vi "Check_bandejas.vi"(8 "error in (no error)":errorcluster, 10 "BANDEJA ORIGEN":T2(ring), 11 "BANDEJA DESTINO":T2(ring)) -> (0 "error out":errorcluster, 2 "States_main":T1, 3 "Datos incorrectos":bool)   [LabVIEW 2019]
uses:
  TYPE'S DEF/Estados_TRASPASO.ctl
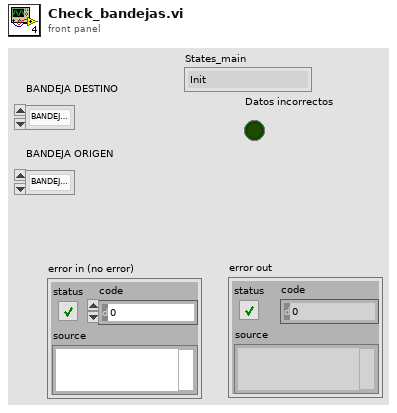
[diagram p1: front panel]
types:
  T1 = typedef "Estados_TRASPASO.ctl" = enum16{"Init", "Wait for Event", "Init refs", "Init com", "Config estacion", "Introducir valores traspaso", "Home", "Ping_Arduino", "Esperar fin movimiento", "Enviar_config_test", "Actualizar valores", "Final traspaso?", "Terminar", "Exit", "Error?"}
  T2 = enum16{"BANDEJA ENTRADA", "BANDEJA OK", "BANDEJA NOK"}
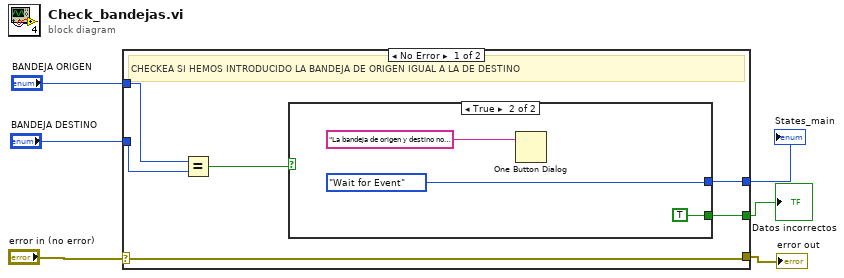
[diagram p0: block diagram]
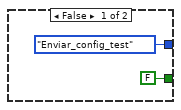
[diagram p2: hidden frame]
diagram:
  n1 = case shown="No Error" "error in (no error)" {
    selector: "error in (no error)" -> [w7 w18]
    tunnel: "BANDEJA DESTINO" -> [w12 _]
    tunnel: "BANDEJA ORIGEN" -> [w11 _]
    tunnel: [w9 _] -> w4
    tunnel: [w8 _] -> w3
    tunnel: [w7 w18] -> w1
    frame No Error {
      # "CHECKEA SI HEMOS INTRODUCIDO LA BANDEJA DE ORIGEN IGUAL A LA DE DESTINO"
      n2 = Equal?(x=w11, y=w12) -> (x = y?=w10:bool)
      n3 = case shown="True" w10 {
        tunnel: [FALSE ("Datos incorrectos") TRUE ("Datos incorrectos")] -> w9
        tunnel: [Estados_TRASPASO."Enviar_config_test" ("States_main") Estados_TRASPASO."Wait for Event" ("States_main")] -> w8
        frame False {
        }
        frame True {
          n4 = One Button Dialog(message="La bandeja de origen y destino no pueden ser iguales.") -> ()  [unwired: 1 in, 1 out]
        }
      }
    }
    frame Error {
    }
  }
  "Datos incorrectos" <- w4
  "States_main" <- w3
  "error out" <- w1
